vi "dfd_Get Narrowband Filter Response.vi"(4 "phase view":T1, 6 "fs in [Hz]":dbl=1.0, 7 "# freq bins":i32=512, 8 "error in (no error)":errorcluster, 9 "dB on? (T)":bool=TRUE, 11 "narrowband filter in":T2 {"multirate filters"."mMRate_SumWl" min=1 max=32 step=1; "multirate filters"."mMRate_InputIwl" min=1 max=32 step=1; "multirate filters"."mMRate_GainWl" min=1 max=32 step=1; "multirate filters"."mMRate_OutputWl" min=1 max=32 step=1; "multirate filters"."mMRate_InputWl" min=1 max=32 step=1; "multirate filters"."mMRate_CoefWl" min=1 max=32 step=1; "multirate filters"."mMRate_Mode" items=["Default"=-1, "No Rate Change"=0, "Interpolation"=1, "Decimation"=2, "Interpolated"=3, "Rational"=4]}) -> (0 "error out":errorcluster, 2 "phase response":cluster{"f0":dbl, "df":dbl, "phase":dbl[]} {"df" format="%.2f"; "f0" format="%.2f"; "phase" format="%.2f"}, 3 "magnitude response":cluster{"f0":dbl, "df":dbl, "magnitude":dbl[]} {"df" format="%.2f"; "f0" format="%.2f"; "magnitude" format="%.2f"})   [LabVIEW 2017, in "NI_DigFilterLicensed.lvlib"]
uses:
  <vilib>/addons/Digital Filter Design/NI_DigFilterLicensed.lvlib
  <vilib>/addons/Digital Filter Design/_Objects.llb/DFD Narrowband Filter Obj.ctl
  <vilib>/addons/Digital Filter Design/_Objects.llb/DFD Multirate Filter Obj.ctl
  <vilib>/addons/Digital Filter Design/_Objects.llb/DFD Multirate Mode.ctl
  <vilib>/addons/Digital Filter Design/_Objects.llb/DFD Coef Norm Type.ctl
  <vilib>/addons/Digital Filter Design/_Objects.llb/DFD Round-off Mode.ctl
  <vilib>/addons/Digital Filter Design/_Objects.llb/DFD FXP MRate Multiply Mode.ctl
  <vilib>/addons/Digital Filter Design/_Objects.llb/DFD Phase Setting.ctl
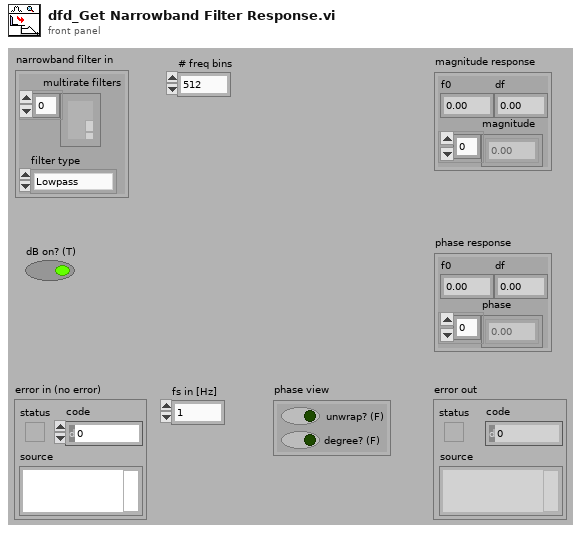
[diagram p1: front panel]
types:
  T1 = typedef "NI_DigFilterLicensed.lvlib/DFD Phase Setting.ctl" = cluster{"unwrap? (F)":bool, "degree? (F)":bool}
  T2 = typedef "NI_DigFilterLicensed.lvlib/DFD Narrowband Filter Obj.ctl" = cluster{"multirate filters":T3[], "filter type":enum32{"Lowpass", "Highpass", "Bandpass", "Bandstop", "Wideband-Lowpass", "Wideband-Highpass"}}
  T3 = typedef "NI_DigFilterLicensed.lvlib/DFD Multirate Filter Obj.ctl" = cluster{"mMRate_Structure":enum16{"CIC", "FIR", "IIR", "Lattice"}, "mMRate_Mode":T4, "mMRate_Factor":i32, "mMRate_FIRParams":cluster{"mMRate_FIR_H":dbl[], "mMRate_FIR_IsNyquist?":bool, "mMRate_FIR_IsSymmetric?":bool}, "mMRate_CICParams":cluster{"mMRate_CIC_#Stage":i32, "mMRate_CIC_Lag":i32, "mMRate_CIC_Type":enum16{"Lowpass", "Highpass"}}, "mMRate_Order":i32, "mMRate_Version":string, "mMRate_Comments":string, "mMRate_RationalFactor":cluster{"mMRate_L":i32, "mMRate_M":i32}, "mMRate_Fs":dbl, "mMRate_Quantized?":bool, "mMRate_QFilterGain":dbl, "mMRate_CoefWl":i16, "mMRate_Scaling":cluster{"mMRate_ScaleByPowerOf2?":bool, "mMRate_ScaleType":T5}, "mMRate_InputWl":i16, "mMRate_OutputWl":i16, "mMRate_OutputMode":T6, "mMRate_MultMode":T7, "mMRate_BitPruning":bool, "mMRate_GainWl":i16, "mMRate_OutputFwl":i16, "mMRate_SumIwl":i16, "mMRate_InputIwl ":i16, "mMRate_SumWl":i16, "mMRate_CoefIwl":i16}
  T4 = typedef "NI_DigFilterLicensed.lvlib/DFD Multirate Mode.ctl" = i16
  T5 = typedef "NI_DigFilterLicensed.lvlib/DFD Coef Norm Type.ctl" = enum16{"No Norm", "Time Domain 1-Norm", "Time Domain 2-Norm", "Time Domain Inf-Norm"}
  T6 = typedef "NI_DigFilterLicensed.lvlib/DFD Round-off Mode.ctl" = enum16{"Nearest", "Truncation"}
  T7 = typedef "NI_DigFilterLicensed.lvlib/DFD FXP MRate Multiply Mode.ctl" = enum16{"Truncated", "Full"}
  T8 = enum32{"Lowpass", "Highpass", "Bandpass", "Bandstop", "Wideband-Lowpass", "Wideband-Highpass"}
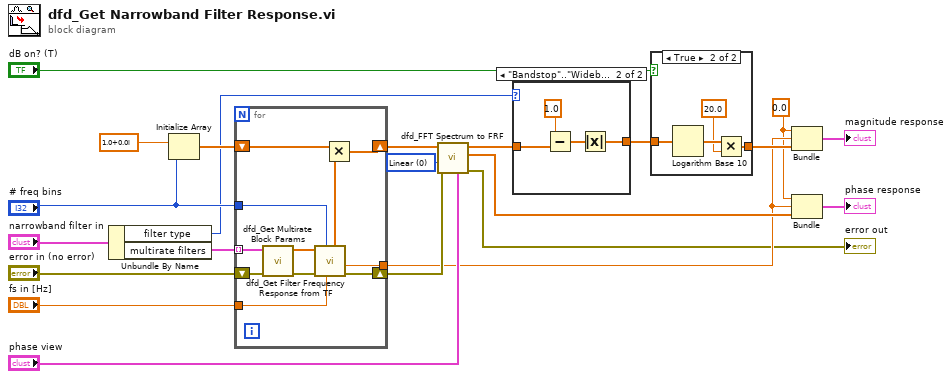
[diagram p0: block diagram]
diagram:
  w1 = u16 0 items=["Linear", "dB", "Zero phase"] ("magnitude")
  w5 = 0.0
  n1 = Unbundle By Name("narrowband filter in") -> ("filter type"=w12:T8, "multirate filters"=w21:T3[])
  n2 = Initialize Array(cdb 1.0+0.0i ("element"), "# freq bins") -> (w17:cdb[])
  n3 = for {
    shift-right: [w29] -> w14
    shift-left: "error in (no error)" -> [w32]
    tunnel: w21 -> [w33] mode=indexing
    tunnel: "fs in [Hz]" -> [w28]
    tunnel: "# freq bins" -> [w27]
    shift-right: [w24] -> w15
    shift-left: w17 -> [w26]
    tunnel: [w23] -> w6
    n4 = call <vilib>:"dfd_Get Multirate Block Params.vi"("error in (no error)"=w32, "multirate filter in"=w33) -> ("error out"=w31:errorcluster, "FIR"=w30:dbl[])  [unwired: 2 in, 6 out]
    n5 = call <vilib>:"dfd_Get Filter Frequency Response from TF.vi"("fs [Hz]"=w28, "# freq bins (512)"=w27, "error in (no error)"=w31, "num"=w30) -> ("error out"=w29:errorcluster, "df"=w23:dbl, "X(w)"=w25:cdb[])  [unwired: 3 in, 2 out]
    n6 = Multiply(x=w26, y=w25) -> (x*y=w24:cdb[])
  }
  n7 = call <vilib>:"dfd_FFT Spectrum to FRF.vi"("phase view"="phase view", "error in (no error)"=w14, "magnitude"=w1, "FFT {X}"=w15) -> ("error out"=→"error out":errorcluster, "phase"=w7:dbl[], "amplitude"=w11:dbl[])  [unwired: 2 in, 3 out]
  n8 = case shown="\"Bandstop\"..\"Wideband-Highpass\"" w12 {
    tunnel: w11 -> [w34 w38]
    tunnel: [w34 w35] -> w10
    frame "Lowpass".."Bandpass", Default {
    }
    frame "Bandstop".."Wideband-Highpass" {
      n9 = Subtract(x=1.0, y=w38) -> (x-y=w36:dbl[])
      n10 = Absolute Value(x=w36) -> (abs(x)=w35:dbl[])
    }
  }
  n11 = case shown="True" "dB on? (T)" {
    tunnel: w10 -> [w39 w43]
    tunnel: [w39 w41] -> w8
    frame False {
    }
    frame True {
      n12 = Logarithm Base 10(1:w43) -> (0:w42:dbl[])
      n13 = Multiply(x=w42, y=20.0) -> (x*y=w41:dbl[])
    }
  }
  n14 = Bundle(w5, "df"=w6, "amplitude"=w8) -> (→"magnitude response":cluster{dbl, "df":dbl, "amplitude":dbl[]})  [unwired: 1 out]
  n15 = Bundle(w5, "df"=w6, "phase"=w7) -> (→"phase response":cluster{dbl, "df":dbl, "phase":dbl[]})  [unwired: 1 out]
